vi "Mean-STD-CoV.vi"(0 "Data Array":dbl[](array[numeric])) -> (4 "Mean":dbl, 6 "Mean":string, 10 "CoV":dbl, 15 "CoV":string)   [LabVIEW 2021]
uses:
  <vilib>/Analysis/NI_AALBase.lvlib
panel:
  out "STD":string
  out "Standard Deviation":dbl format="%0.2f"
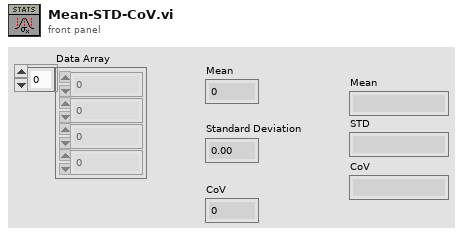
[diagram p1: front panel]
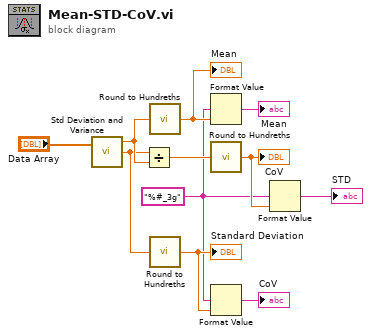
[diagram p0: block diagram]
diagram:
  w1 = "%#_3g" ("format string")
  n1 = call <vilib>:"Std Deviation and Variance.vi"("X"="Data Array") -> ("mean"=w5:dbl, "standard deviation"=w3:dbl)  [unwired: 1 in, 1 out]
  n2 = Divide(x=w3, y=w5) -> (x/y=w4:dbl)
  n3 = call "Round to Hundreths.vi"("Raw"=w5) -> ("Rounded"=w2:dbl)  [unwired: 4 in]
  "Mean" <- w2
  n4 = call "Round to Hundreths.vi"("Raw"=w3) -> ("Rounded"=w7:dbl)  [unwired: 4 in]
  "Standard Deviation" <- w7
  n5 = Format Value(format string=w1, value (0)=w2) -> (output string=→"Mean":string)  [unwired: 1 in]
  n6 = call "Round to Hundreths.vi"("Raw"=w4) -> ("Rounded"=w6:dbl)  [unwired: 4 in]
  "CoV" <- w6
  n7 = Format Value(format string=w1, value (0)=w7) -> (output string=→"CoV":string)  [unwired: 1 in]
  n8 = Format Value(format string=w1, value (0)=w6) -> (output string=→"STD":string)  [unwired: 1 in]
